vi "Generate ConfigFile Path.vi"() -> (0 "ConfigFile path":path)   [LabVIEW 2018, in "FPGA Addon DMA Waveform Status Channel System Tests.lvclass"]
uses:
  FPGA Addon DMA Waveform Status Channel System Tests.lvclass
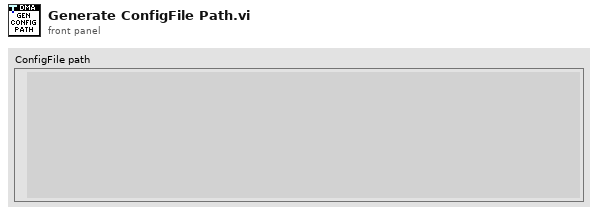
[diagram p1: front panel]
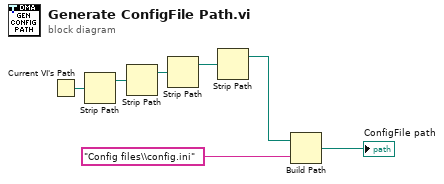
[diagram p0: block diagram]
diagram:
  n1 = Current VI's Path() -> (path=w7:path)
  n2 = Strip Path(path=w7) -> (stripped path=w6:path)  [unwired: 1 out]
  n3 = Strip Path(path=w6) -> (stripped path=w5:path)  [unwired: 1 out]
  n4 = Strip Path(path=w5) -> (stripped path=w2:path)  [unwired: 1 out]
  n5 = Strip Path(path=w2) -> (stripped path=w1:path)  [unwired: 1 out]
  n6 = Build Path(base path=w1, name or relative path="Config files\\config.ini") -> (appended path=→"ConfigFile path":path)
